vi "Histogram2D_Manual.vi"(4 "Properties":T1={"Normalize"=FALSE, "Colormap"={"Map"=enum."Automatic", "Value Min"=nan, "Value Max"=nan, "Scaling"=enum."Default", "Reverse"=FALSE}, "Display"={"Alpha"=nan, "Z Order"=nan}}, 5 "Y Bin Edges":dbl[](array[numeric]), 7 "X Bin Edges":dbl[](array[numeric]), 8 "error in (no error)":errorcluster, 9 "Y Data":dbl[](array[numeric]), 10 "X Data":dbl[](array[numeric]), 11 "Plot ID":T6 format="%x") -> (0 "error out":errorcluster, 3 "Plot ID Out":T6 format="%x")   [LabVIEW 2013, in "Advanced Plotting Toolkit.lvlib"]
doc: "Create a 2D histogram from two data sets in X and Y, visualized as a 2D plane of colored patches. Explicitly specify the locations of the bin edges in X and Y."
uses:
  Advanced Plotting Toolkit.lvlib
  typedefs/PlotID.ctl
  Histogram2DProperties.ctl
  properties/Colormap.ctl
  properties/Colormap_Map.ctl
  properties/Colormap_Scaling.ctl
  properties/Display.ctl
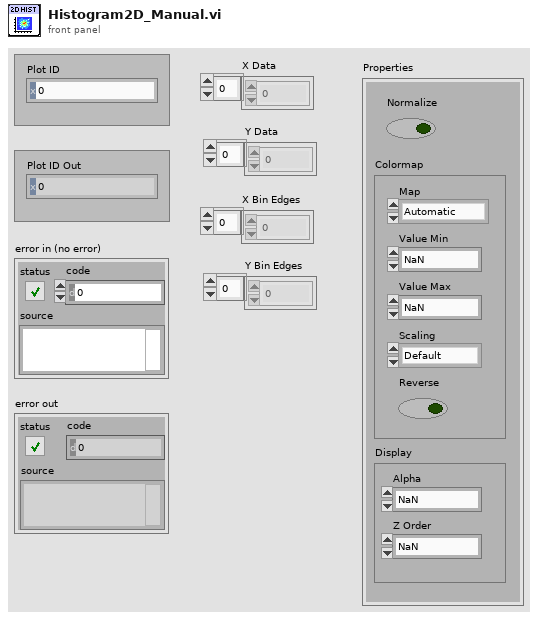
[diagram p1: front panel]
types:
  T1 = typedef "Advanced Plotting Toolkit.lvlib/Histogram2DProperties.ctl" = cluster{"Normalize":bool, "Colormap":T2, "Display":T5}
  T2 = typedef "Advanced Plotting Toolkit.lvlib/Colormap.ctl" = cluster{"Map":T3, "Value Min":dbl, "Value Max":dbl, "Scaling":T4, "Reverse":bool}
  T3 = typedef "Advanced Plotting Toolkit.lvlib/Colormap_Map.ctl" = enum16{"Automatic", "Rainbow", "Hot and Cold", "White-Black", "White-Blue", "White-Green", "White-Red", "Fire", "Water", "Earth", "Air", "Pastel", "Banded", "Stepped"}
  T4 = typedef "Advanced Plotting Toolkit.lvlib/Colormap_Scaling.ctl" = enum16{"Default"}
  T5 = typedef "Advanced Plotting Toolkit.lvlib/Display.ctl" = cluster{"Alpha":dbl, "Z Order":dbl}
  T6 = typedef "Advanced Plotting Toolkit.lvlib/PlotID.ctl" = i32
  T7 = typedef "Advanced Plotting Toolkit.lvlib/KeyValue.ctl" = cluster{"Key":string, "Value":string}
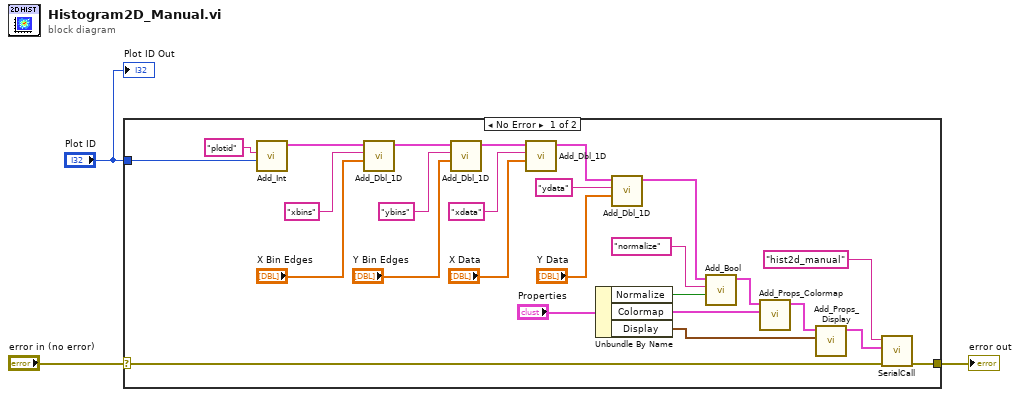
[diagram p0: block diagram]
diagram:
  n1 = case shown="No Error" "error in (no error)" {
    selector: "error in (no error)" -> [w24 w30]
    tunnel: "Plot ID" -> [w29 _]
    tunnel: [w23 w30] -> w1
    frame No Error {
      n2 = call "Add_Int.vi"("Value"=w29, "Key"="plotid") -> ("Keyword Array Out"=w12:T7[])  [unwired: 9 in]
      n3 = call "Add_Dbl_1D.vi"("Value"="X Bin Edges", "Key"="xbins", "Keyword Array"=w12) -> ("Keyword Array Out"=w9:T7[])  [unwired: 8 in]
      n4 = call "Add_Dbl_1D.vi"("Value"="Y Bin Edges", "Key"="ybins", "Keyword Array"=w9) -> ("Keyword Array Out"=w6:T7[])  [unwired: 8 in]
      n5 = call "Add_Dbl_1D.vi"("Value"="X Data", "Key"="xdata", "Keyword Array"=w6) -> ("Keyword Array Out"=w22:T7[])  [unwired: 8 in]
      n6 = Unbundle By Name("Properties") -> ("Normalize"=w16:bool, "Colormap"=w14:T2, "Display"=w13:T5)
      n7 = call "Add_Dbl_1D.vi"("Value"="Y Data", "Key"="ydata", "Keyword Array"=w22) -> ("Keyword Array Out"=w17:T7[])  [unwired: 8 in]
      n8 = call "Add_Bool.vi"("Value"=w16, "Key"="normalize", "Keyword Array"=w17) -> ("Keyword Array Out"=w4:T7[])  [unwired: 8 in]
      n9 = call "Add_Props_Colormap.vi"("Colormap"=w14, "Keyword Array"=w4) -> ("Keyword Array Out"=w15:T7[])  [unwired: 9 in]
      n10 = call "Add_Props_Display.vi"("Display"=w13, "Keyword Array"=w15) -> ("Keyword Array Out"=w5:T7[])  [unwired: 9 in]
      n11 = call "SerialCall.vi"("error in (no error)"=w24, "data"=w5, "Resource"="hist2d_manual") -> ("error out"=w23:errorcluster)  [unwired: 7 in, 1 out]
    }
    frame Error {
    }
  }
  "error out" <- w1
  "Plot ID Out" <- "Plot ID"
